vi "Add Response (Invalid Request).vi"(5 "id value":string, 7 "jsonrpc":string, 8 "error in (no error)":errorcluster, 10 "data":variant, 11 "Server in":refnum<class "JSONRPC Server.lvclass">) -> (0 "error out":errorcluster, 3 "Server out":refnum<class "JSONRPC Server.lvclass">)   [LabVIEW 2015, in "JSONRPC Server.lvclass"]
uses:
  JSONRPC Server.lvclass
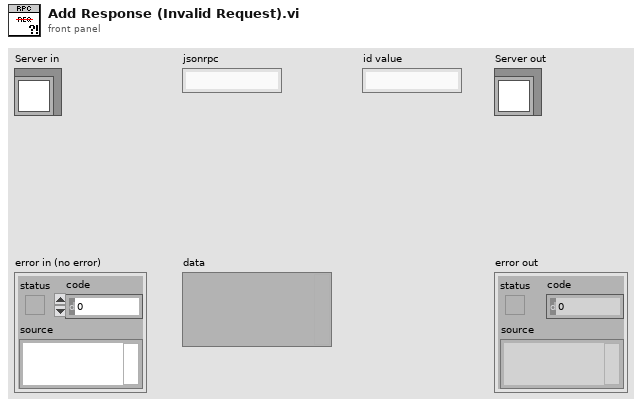
[diagram p1: front panel]
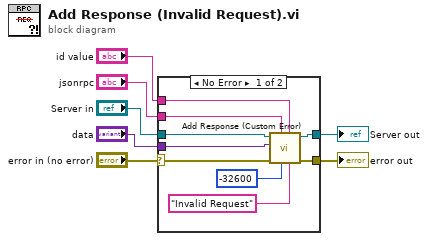
[diagram p0: block diagram]
diagram:
  n1 = case shown="No Error" "error in (no error)" {
    selector: "error in (no error)" -> [w8 w18]
    tunnel: [w9 w18] -> w6
    tunnel: [w15 w17] -> w4
    tunnel: "Server in" -> [w16 w17]
    tunnel: "data" -> [w12 _]
    tunnel: "jsonrpc" -> [w11 _]
    tunnel: "id value" -> [w10 _]
    frame No Error {
      n2 = call "Add Response (Custom Error).vi"("message"="Invalid Request", "id value"=w10, "code"=-32600, "jsonrpc"=w11, "error in (no error)"=w8, "data"=w12, "Server in"=w16) -> ("error out"=w9:errorcluster, "Server out"=w15:refnum<class "JSONRPC Server.lvclass">)  [unwired: 3 in]
    }
    frame Error {
    }
  }
  "error out" <- w6
  "Server out" <- w4
